vi "band to color converter.vi"(2 "Digit":T1) -> (6 "Color":u32(colorbox))   [LabVIEW 2018]
uses:
  significant digit--control.ctl
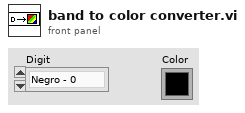
[diagram p1: front panel]
types:
  T1 = typedef "significant digit--control.ctl" = enum16{"Negro - 0", "Marrón - 1", "Rojo - 2", "Naranja - 3", "Amarillo - 4", "Verde - 5", "Azul - 6", "Violeta - 7", "Gris - 8", "Blanco - 9"}
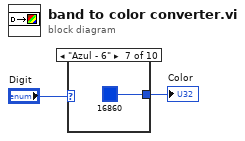
[diagram p0: block diagram]
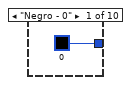
[diagram p2: hidden frame]
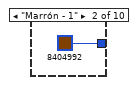
[diagram p3: hidden frame]
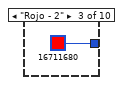
[diagram p4: hidden frame]
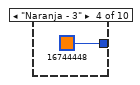
[diagram p5: hidden frame]
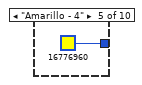
[diagram p6: hidden frame]
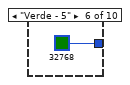
[diagram p7: hidden frame]
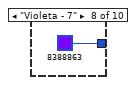
[diagram p8: hidden frame]
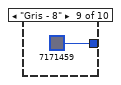
[diagram p9: hidden frame]
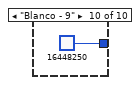
[diagram p10: hidden frame]
diagram:
  n1 = case shown="\"Azul - 6\"" "Digit" {
    tunnel: [u32 0 u32 8404992 u32 16711680 u32 16744448 u32 16776960 u32 32768 u32 16860 u32 8388863 u32 7171459 u32 16448250] -> w1
    frame "Negro - 0" {
    }
    frame "Marrón - 1" {
    }
    frame "Rojo - 2" {
    }
    frame "Naranja - 3" {
    }
    frame "Amarillo - 4" {
    }
    frame "Verde - 5" {
    }
    frame "Azul - 6" {
    }
    frame "Violeta - 7" {
    }
    frame "Gris - 8" {
    }
    frame "Blanco - 9" {
    }
  }
  "Color" <- w1
